vi "Main.vi"(11 "Module Admin":refnum<class "Delacor_lib_QMH_Module Admin.lvclass">) -> ()   [LabVIEW 2020, in "MainUI.lvlib"]
doc: "This template is based off of the Queued Message Handler design pattern and the Queued Message Handler project template that ships with LabVIEW.\n\nThe main difference is that the queue is private to this module and communication between modules is performed via Broadcast and Request events.\n\nRequest events are wrapped in public API methods and are handled in the Event Handling Loop (EHL) of this VI. Any module can register for Broadcast events sent by this module. The EHL generates messages based on user interface actions.\n\nThe Message Handling Loop (MHL) processes messages generated by the EHL, or by other messages. The messages are string values, so new messages can be added easily to the Message Cases case structure in the MHL. Each message cluster can also provide an optional value for Message Data, which is a variant that can be converted to whatever message-specific data is required.\n_____\nBased on Delacor QMH Project Template 4.0.0.47.\n_____\nBased on Delacor QMH Project Template 5.0.0.82."
uses:
  MainUI.lvlib
  <vilib>/Delacor/Delacor QMH/Libraries/Module Admin_class/Delacor_lib_QMH_Module Admin.lvclass
  Module Data--cluster.ctl
  Stop Argument--cluster.ctl
  <vilib>/Delacor/Delacor QMH/Libraries/Message Queue_class/Delacor_lib_QMH_Message Queue.lvclass/Delacor_lib_QMH_Message Queue.ctl
  <vilib>/Delacor/Delacor QMH/Libraries/Module Admin_class/Delacor_lib_QMH_Module Admin.lvclass/Delacor_lib_QMH_Module Admin.ctl
  <vilib>/Delacor/Delacor QMH/Libraries/Message Queue_class/Delacor_lib_QMH_Enqueue Message (Single).vi
  <vilib>/Delacor/Delacor QMH/Libraries/Module Admin_class/Delacor_lib_QMH_Get External Launch.vi
  <vilib>/Waveform/WDTOps.llb/WDT Get XY Value DBL.vi
  <vilib>/Utility/error.llb/Error Cluster From Error Code.vi
  <vilib>/ErrorRing/Error Ring.xnode
  <vilib>/Delacor/Delacor QMH/Libraries/Message Queue_class/Delacor_lib_QMH_Message Queue.lvclass
  Settings Editor/Settings Editor.lvlib
  Acquisition/GetTemperature.lvlib
  Logger/FileLogging.lvlib
panel:
  out "Data":waveform(dbl)[](graph)
  out "Log File Base Path":path
  out "Thermocouple Channel":refnum<k21>
  out "Units\nUnits":i32(ring) items=["degC", "degF", "kelvin", "raw"]
  out "Temperature":dbl
  out "Time Stamp":timestamp
  out "Status":string
  out "Calibrated?":bool
  in  "Calibrate":bool
  in  "Settings":bool
  in  "Start":bool
  in  "Stop":bool
  out "Logger Running?":bool
  out "Settings Editor Running?":bool
  out "Acquisition Running?":bool
  out "error out":errorcluster
  out "version":string
  # "Thermocouple Device Channel Logging"
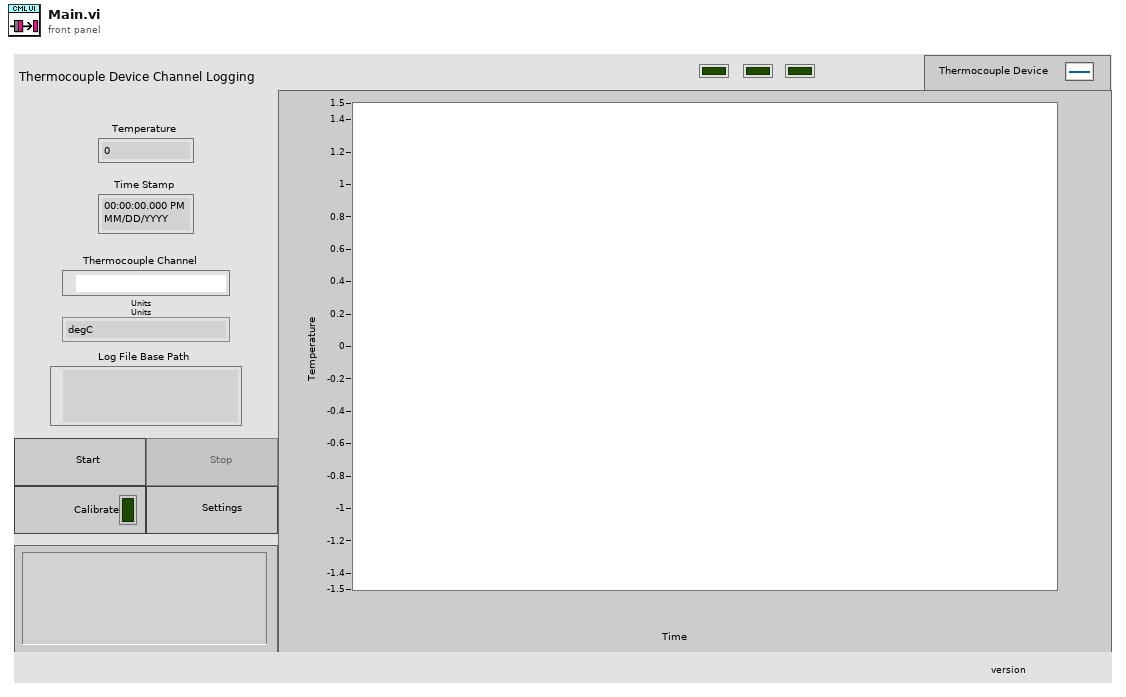
[diagram p1: front panel]
types:
  T1 = typedef "MainUI.lvlib/Request Events--cluster.ctl" = cluster{"Stop Module":refnum<user-event>, "Show Panel":refnum<user-event>, "Hide Panel":refnum<user-event>, "Get Module Execution Status":refnum<user-event>, "Show Diagram":refnum<user-event>}
  T2 = typedef "Settings Editor.lvlib/Broadcast Events--cluster.ctl" = cluster{"Module Did Init":refnum<user-event>, "Status Updated":refnum<user-event>, "Error Reported":refnum<user-event>, "Module Did Stop":refnum<user-event>, "Update Module Execution Status":refnum<user-event>, "Application Settings Updated":refnum<user-event>}
  T3 = typedef "GetTemperature.lvlib/Broadcast Events--cluster.ctl" = cluster{"Module Did Init":refnum<user-event>, "Status Updated":refnum<user-event>, "Error Reported":refnum<user-event>, "Module Did Stop":refnum<user-event>, "Update Module Execution Status":refnum<user-event>, "Acquisition Started":refnum<user-event>, "Acquisition Stopped":refnum<user-event>, "Data Updated":refnum<user-event>, "Device Calibrated":refnum<user-event>}
  T4 = typedef "FileLogging.lvlib/Broadcast Events--cluster.ctl" = cluster{"Module Did Init":refnum<user-event>, "Status Updated":refnum<user-event>, "Error Reported":refnum<user-event>, "Module Did Stop":refnum<user-event>, "Update Module Execution Status":refnum<user-event>, "Logging Stopped":refnum<user-event>, "File Initialized":refnum<user-event>}
  T5 = typedef "MainUI.lvlib/Module Data--cluster.ctl" = cluster{"Status":string, "Measurement UI Controls":cluster{"Start Ref":refnum<vi>, "Stop Ref":refnum<vi>, "Settings Ref":refnum<vi>, "Status Ref":refnum<vi>, "Data Ref":refnum<vi>}}
  T6 = enum32{"invalid lock state", "Not Locked", "Locked (No Password)", "Password-protected"}
  T7 = typedef "MainUI.lvlib/Stop Argument--cluster.ctl" = cluster{"Origin":string, "Exit via Stop Module Req?":bool, "Wait for Module to stop?":bool}
  T8 = enum32{"Invalid", "Standard", "Closed", "Hidden", "Minimized", "Maximized"}
  T9 = typedef "Settings Editor.lvlib/Update Application Settings (Reply Payload)--cluster.ctl" = cluster{"Settings":T10, "Update Settings_error":errorcluster}
  T10 = typedef "Settings Editor.lvlib/Settings--cluster.ctl" = cluster{"Log File Base Path":path, "Analog Input Channel":refnum<k21>, "Units":i32}
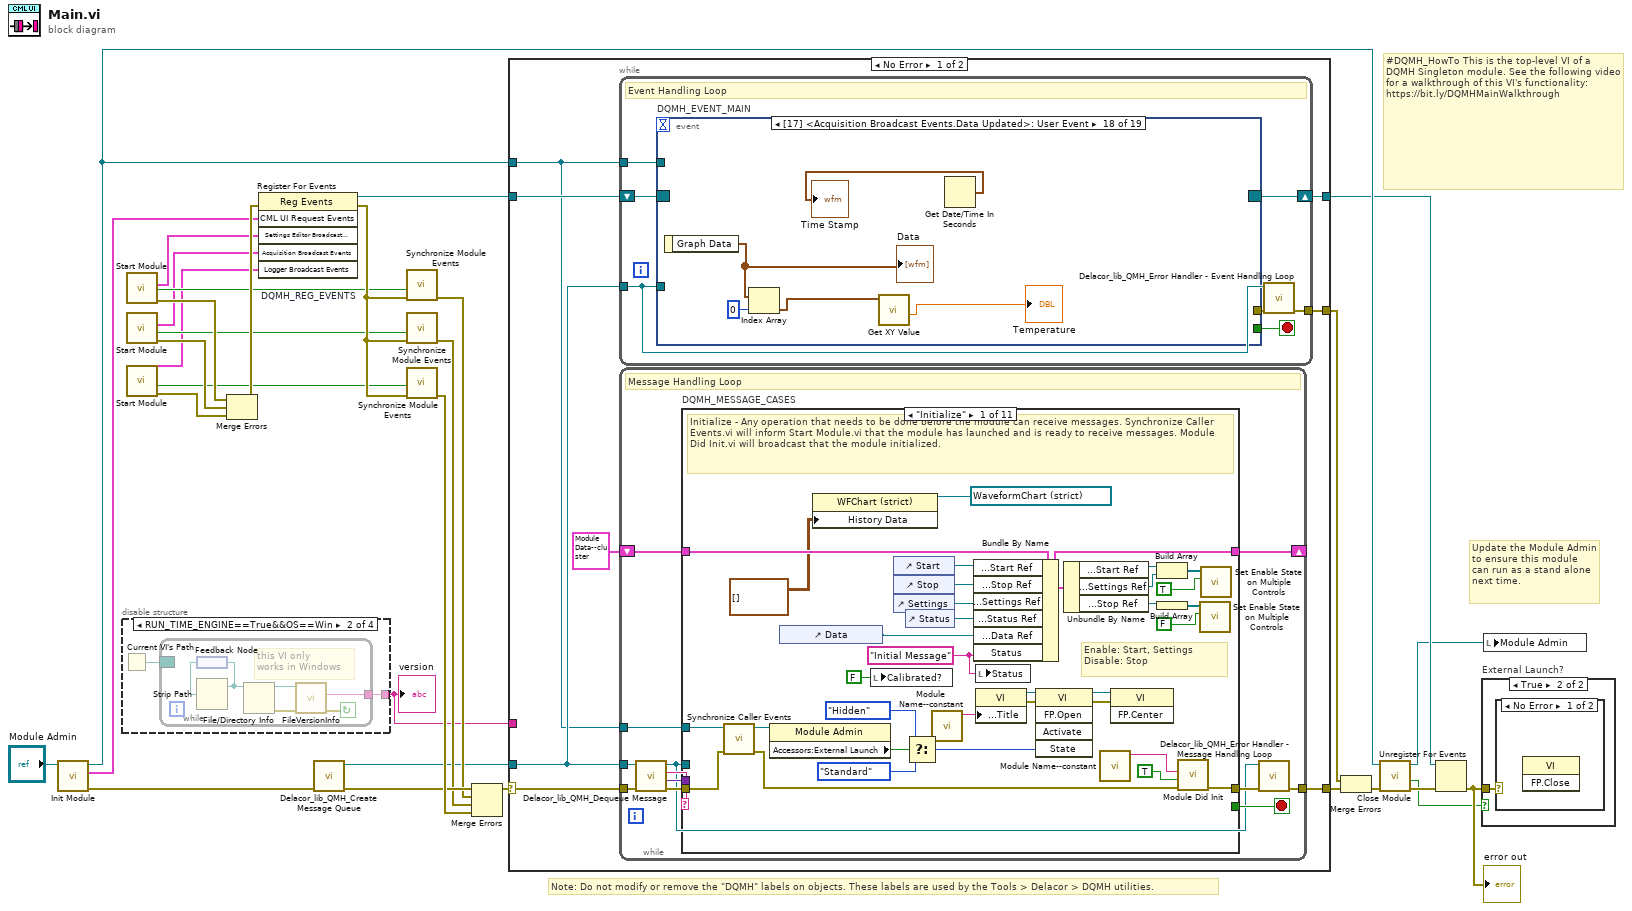
[diagram p0: block diagram]
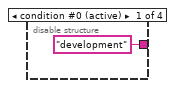
[diagram p2: hidden frame]
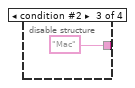
[diagram p3: hidden frame]
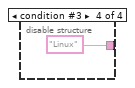
[diagram p4: hidden frame]
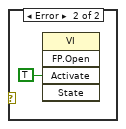
[diagram p6: hidden frame]
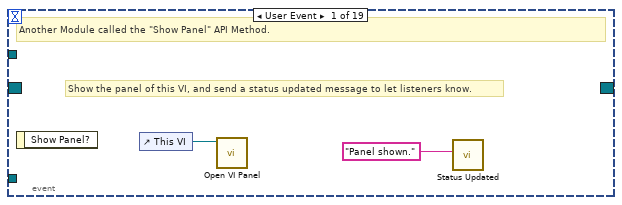
[diagram p7: hidden frame]
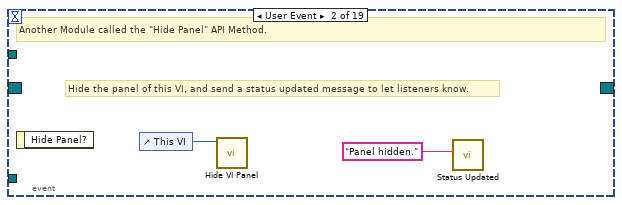
[diagram p8: hidden frame]
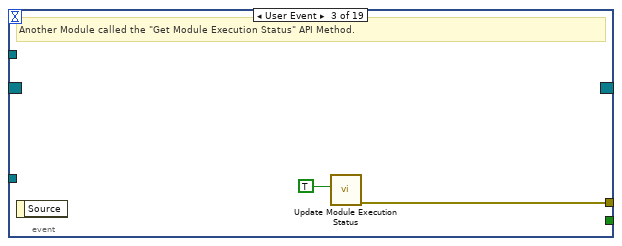
[diagram p9: hidden frame]
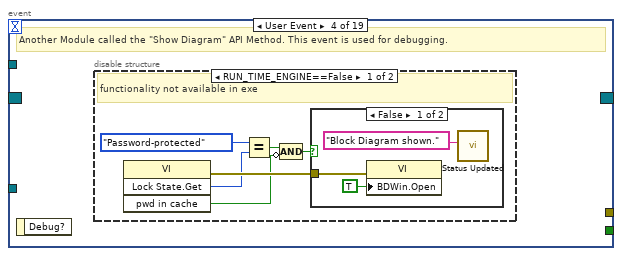
[diagram p10: hidden frame]
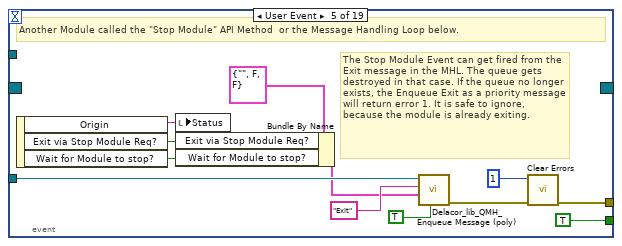
[diagram p13: hidden frame]
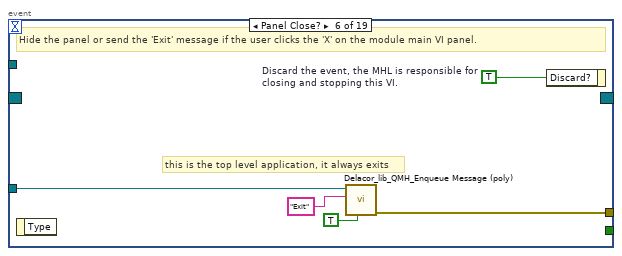
[diagram p14: hidden frame]
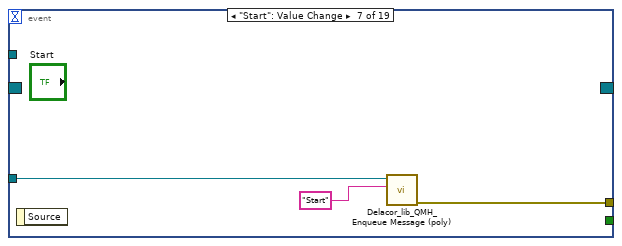
[diagram p15: hidden frame]
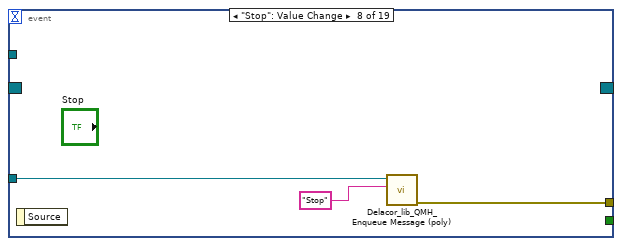
[diagram p16: hidden frame]
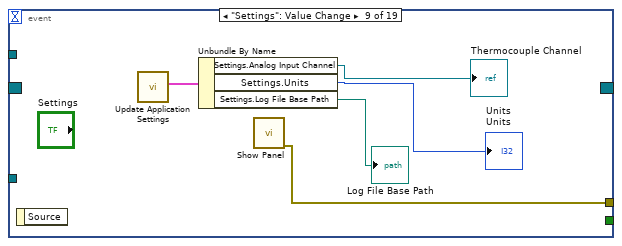
[diagram p17: hidden frame]
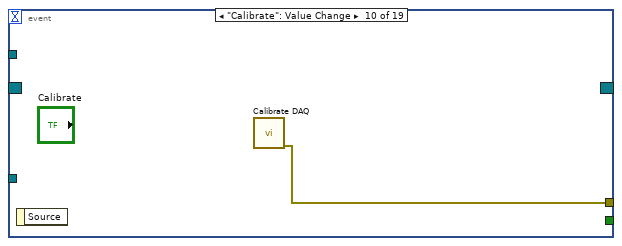
[diagram p18: hidden frame]
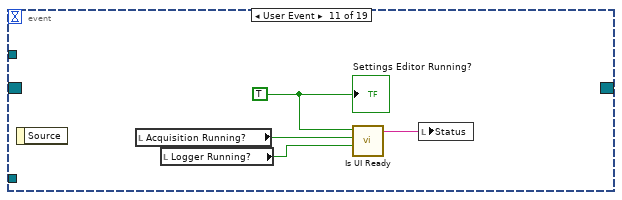
[diagram p19: hidden frame]
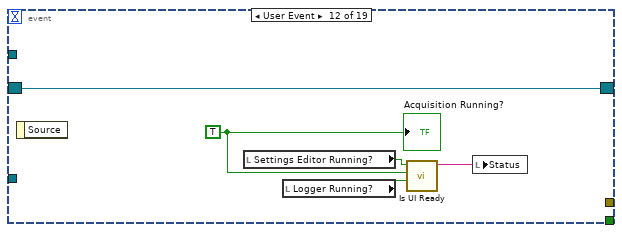
[diagram p20: hidden frame]
diagram:
  # "#DQMH_HowTo This is the top-level VI of a DQMH Singleton module. See the following video for a walkthrough of this VI's functionality: https://bit.ly/DQMHMainWalkthrough"
  # "Note: Do not modify or remove the \"DQMH\" labels on objects. These labels are used by the Tools > Delacor > DQMH utilities."
  # "Update the Module Admin to ensure this module can run as a stand alone next time."
  n1 = call "Init Module.vi"("Singleton Module Admin in"="Module Admin") -> ("error out"=w29:errorcluster, "CML UI Request Events"=w12:T1, "Singleton Module Admin out"=w15:refnum<class "Delacor_lib_QMH_Module Admin.lvclass">)  [unwired: 8 in]
  n2 = disable-structure "Conditional Disable Structure" shown="RUN_TIME_ENGINE==True&&OS==Win" {
    disable-tunnel: ["development" w33 "Mac" "Linux"] -> w1
    frame condition #0 (active) {
    }
    frame condition #1 {
      n3 = Current VI's Path() -> (path=w34:path)
      n4 = while {
        border: w34 -> [_]
        tunnel: [w35] -> w33
        stop <- w39 continue-if-true
        # "this VI only \nworks in Windows"
        n5 = feedback #1() -> (w38:path)
        n6 = Strip Path(path=w38) -> (stripped path=w37:path)  [unwired: 1 out]
        n7 = feedback-in #1(w37) -> ()
        n8 = File/Directory Info(path=w37) -> (path out=w36:path, error out=w40:errorcluster)  [unwired: 1 in, 5 out]
        n9 = call <vilib>:"FileVersionInfo.vi"("error in (no error)"=w40, "Application Path in"=w36) -> ("error out"=w39:errorcluster, "File Version Info"=w35:string)  [unwired: 6 in, 2 out]
      }
    }
    frame condition #2 {
    }
    frame condition #3 {
    }
  }
  "version" <- w1
  n10 = call "Start Module.vi"() -> ("error out"=w20:errorcluster, "Wait for Event Sync?"=w7:bool, "Settings Editor Broadcast Events"=w6:T2)  [unwired: 8 in, 1 out]
  n11 = call "Start Module.vi"() -> ("error out"=w19:errorcluster, "Wait for Event Sync?"=w4:bool, "Acquisition Broadcast Events"=w5:T3)  [unwired: 8 in, 1 out]
  n12 = call "Start Module.vi"() -> ("error out"=w18:errorcluster, "Wait for Event Sync?"=w2:bool, "Logger Broadcast Events"=w3:T4)  [unwired: 8 in, 1 out]
  n13 = Merge Errors(w20, w19, w18) -> (w17:errorcluster)
  n14 = register-events "DQMH_REG_EVENTS"(error in=w17, w12, w6, w5, w3) -> (reference out=w13:refnum<event-registration>, error out=w16:errorcluster)  [unwired: 1 in]
  n15 = call <vilib>:"Delacor_lib_QMH_Create Message Queue.vi"("error in (no error)"=w29) -> ("error out"=w24:errorcluster, "Message Queue"=w11:refnum<class "Delacor_lib_QMH_Message Queue.lvclass">)  [unwired: 9 in]
  n16 = call "Synchronize Module Events.vi"("error in (no error)"=w16, "Wait for Event Sync?"=w7) -> ("error out"=w22:errorcluster)  [unwired: 9 in]
  n17 = call "Synchronize Module Events.vi"("error in (no error)"=w16, "Wait for Event Sync?"=w4) -> ("error out"=w21:errorcluster)  [unwired: 9 in]
  n18 = call "Synchronize Module Events.vi"("error in (no error)"=w16, "Wait for Event Sync?"=w2) -> ("error out"=w31:errorcluster)  [unwired: 9 in]
  n19 = Merge Errors(w24, w22, w21, w31) -> (w23:errorcluster)
  n20 = case shown="No Error" w23 {
    selector: w23 -> [w48 w263]
    tunnel: [w50 w262] -> w30
    tunnel: [w47 w271] -> w14
    tunnel: w13 -> [w45 w271]
    tunnel: w11 -> [w44 w264]
    tunnel: [w49 _] -> w27
    tunnel: w15 -> [w43 w267]
    tunnel: w1 -> [_ _]
    frame No Error {
      n21 = while {
        tunnel: w44 -> [w51]
        shift-right: [w54] -> w47
        shift-left: w45 -> [w55]
        tunnel: [w56] -> w49
        tunnel: w43 -> [w52]
        stop <- w53 stop-if-true
        # "Event Handling Loop"
        n22 = event "DQMH_EVENT_MAIN" shown="[17] <Acquisition Broadcast Events.Data Updated>: User Event" {
          selector: w55 -> [_ _ _ _ _ _ _ _ _ _ _ w110 _ _ _ _ _ _ _]
          dyn-events: [_ _ _ _ _ _ _ _ _ _ _ w110 _ _ _ _ _ _ _] -> w54
          timeout: _ -> [_ _ _ _ _ _ _ _ _ _ _ _ _ _ _ _ _ _ _]
          tunnel: [_ _ _ _ TRUE ("Discard?") _ _ _ _ _ _ _ _ _ _ _ _ _ _] -> w53
          tunnel: w51 -> [_ _ _ _ w80 w87 w90 w93 _ _ _ _ _ _ _ w122 w124 _ _]
          tunnel: [_ _ w63 _ w83 w89 w92 w95 w100 w101 _ _ _ _ w120 _ _ _ _] -> w57
          tunnel: w52 -> [_ _ _ _ _ _ _ _ _ _ _ _ _ _ _ _ _ _ _]
          event User Event {
            # "Show the panel of this VI, and send a status updated message to let listeners know."
            # "Another Module called the \"Show Panel\" API Method."
            n23 = event-data() -> ()  [unwired: 1 in, 1 out]
            n24 = control-ref of="This VI"() -> (w59:refnum<vi>)
            n25 = call "Open VI Panel.vi"("VI"=w59) -> ()  [unwired: 10 in, 1 out]
            n26 = call "Status Updated.vi"("Status"="Panel shown." ("format string")) -> ()  [unwired: 10 in, 1 out]
          }
          event User Event {
            # "Hide the panel of this VI, and send a status updated message to let listeners know."
            # "Another Module called the \"Hide Panel\" API Method."
            n27 = event-data() -> ()  [unwired: 1 in, 1 out]
            n28 = control-ref of="This VI"() -> (w61:refnum<vi>)
            n29 = call "Hide VI Panel.vi"("VI"=w61) -> ()  [unwired: 10 in, 1 out]
            n30 = call "Status Updated.vi"("Status"="Panel hidden." ("format string")) -> ()  [unwired: 10 in, 1 out]
          }
          event User Event {
            # "Another Module called the \"Get Module Execution Status\" API Method."
            n31 = event-data() -> ()  [unwired: 1 in, 1 out]
            n32 = call "Update Module Execution Status.vi"("Running?"=TRUE) -> ("error out"=w63:errorcluster)  [unwired: 10 in]
          }
          event User Event {
            # "Another Module called the \"Show Diagram\" API Method. This event is used for debugging."
            n33 = event-data() -> ()  [unwired: 1 in, 1 out]
            n34 = disable-structure shown="RUN_TIME_ENGINE==False" {
              frame condition #0 (active) {
                # "functionality not available in exe"
                n35 = invoke on="Invoke Node" class="VI" method="Lock State.Get"() -> (error out=w69:errorcluster, "Get Lock State"=w68:T6, "pwd in cache"=w65:bool)  [unwired: 4 in, 1 out]
                n36 = Equal?(x=T6."Password-protected", y=w68) -> (x = y?=w66:bool)
                n37 = Compound Arithmetic op=AND(w66, invert w65) -> (w64:bool)
                n38 = case shown="False" w64 {
                  tunnel: w69 -> [w72 _]
                  frame False {
                    n39 = property on="Property Node" class="VI"(error in=w72, "BDWin.Open"=TRUE ("Block Diagram Window:Open")) -> ()  [unwired: 1 in, 2 out]
                    n40 = call "Status Updated.vi"("Status"="Block Diagram shown." ("format string")) -> ()  [unwired: 10 in, 1 out]
                  }
                  frame True {
                    # "Password-protected VI, and the password is not in the cache. Do not show the diagram."
                  }
                }
              }
              frame condition #1 {
              }
            }
          }
          event User Event {
            # "The Stop Module Event can get fired from the Exit message in the MHL. The queue gets destroyed in that case. If the queue no longer exists, the Enqueue Exit as a priority message will return error 1. It is safe to ignore, because the module is already exiting."
            # "Another Module called the \"Stop Module\" API Method  or the Message Handling Loop below."
            n41 = event-data() -> ("Origin"=w79:string, "Exit via Stop Module Req?"=w75:bool, "Wait for Module to stop?"=w74:bool)  [unwired: 1 in]
            n42 = local write "Status"(w79) -> ()
            n43 = Bundle By Name(cluster=T7 {"Origin"="", "Exit via Stop Module Req?"=FALSE, "Wait for Module to stop?"=FALSE} ("Stop Argument"), "Exit via Stop Module Req?"=w75, "Wait for Module to stop?"=w74) -> (w73:T7)
            n44 = call-poly <vilib>:"Delacor_lib_QMH_Enqueue Message (poly).vi"("Priority Message? (F)"=TRUE, "Message Data"=w73, "Message"="Exit", "Message Queue in"=w80) -> ("error out"=w84:errorcluster)  [unwired: 6 in, 1 out]
            n45 = call <vilib>:"Clear Errors.vi"("error in (no error)"=w84, "specific error code to clear (0: all)"=1) -> ("error out"=w83:errorcluster)  [unwired: 4 in, 1 out]
          }
          event Panel Close? {
            w88 = TRUE  # Discard the event, the MHL is responsible for closing and stopping this VI.
            # "this is the top level application, it always exits"
            # "Hide the panel or send the 'Exit' message if the user clicks the 'X' on the module main VI panel."
            n46 = event-data() -> ()  [unwired: 1 in, 1 out]
            n47 = call-poly <vilib>:"Delacor_lib_QMH_Enqueue Message (poly).vi"("Priority Message? (F)"=TRUE, "Message"="Exit", "Message Queue in"=w87) -> ("error out"=w89:errorcluster)  [unwired: 7 in, 1 out]
            n48 = event-data ("Event Filter Node")("Discard?"=w88) -> ()  [unwired: 1 in, 1 out]
          }
          event "Start": Value Change {
            n49 = event-data() -> ()  [unwired: 1 in, 1 out]
            n50 = call-poly <vilib>:"Delacor_lib_QMH_Enqueue Message (poly).vi"("Message"="Start", "Message Queue in"=w90) -> ("error out"=w92:errorcluster)  [unwired: 8 in, 1 out]
          }
          event "Stop": Value Change {
            n51 = event-data() -> ()  [unwired: 1 in, 1 out]
            n52 = call-poly <vilib>:"Delacor_lib_QMH_Enqueue Message (poly).vi"("Message"="Stop", "Message Queue in"=w93) -> ("error out"=w95:errorcluster)  [unwired: 8 in, 1 out]
          }
          event "Settings": Value Change {
            n53 = event-data() -> ()  [unwired: 1 in, 1 out]
            n54 = call "Update Application Settings.vi"() -> ("Reply Payload"=w99:T9)  [unwired: 9 in, 2 out]
            n55 = Unbundle By Name(w99) -> ("Settings.Analog Input Channel"=→"Thermocouple Channel":refnum<k21>, "Settings.Units"=→"Units\nUnits":i32, "Settings.Log File Base Path"=→"Log File Base Path":path)
            n56 = call "Show Panel.vi"() -> ("error out"=w100:errorcluster)  [unwired: 11 in]
          }
          event "Calibrate": Value Change {
            n57 = event-data() -> ()  [unwired: 1 in, 1 out]
            n58 = call "Calibrate DAQ.vi"() -> ("error out"=w101:errorcluster)  [unwired: 11 in]
          }
          event User Event {
            w103 = TRUE ("Settings Editor Running?")
            n59 = event-data() -> ()  [unwired: 1 in, 1 out]
            n60 = local read "Acquisition Running?"() -> (w105:bool)
            n61 = local read "Logger Running?"() -> (w104:bool)
            n62 = call "Is UI Ready.vi"("Logger Running?"=w104, "Acquisition Running?"=w105, "Settings Editor Running?"=w103) -> ("Status"=w102:string)  [unwired: 8 in]
            n63 = local write "Status"(w102) -> ()
            "Settings Editor Running?" <- w103
          }
          event User Event {
            w108 = TRUE ("Acquisition Running?")
            n64 = event-data() -> ()  [unwired: 1 in, 1 out]
            n65 = local read "Settings Editor Running?"() -> (w107:bool)
            n66 = local read "Logger Running?"() -> (w106:bool)
            n67 = call "Is UI Ready.vi"("Logger Running?"=w106, "Acquisition Running?"=w108, "Settings Editor Running?"=w107) -> ("Status"=w109:string)  [unwired: 8 in]
            n68 = local write "Status"(w109) -> ()
            "Acquisition Running?" <- w108
          }
          event User Event {
            w113 = TRUE ("Logger Running?")
            n69 = event-data() -> ()  [unwired: 1 in, 1 out]
            n70 = local read "Settings Editor Running?"() -> (w112:bool)
            n71 = local read "Acquisition Running?"() -> (w111:bool)
            n72 = call "Is UI Ready.vi"("Logger Running?"=w113, "Acquisition Running?"=w111, "Settings Editor Running?"=w112) -> ("Status"=w114:string)  [unwired: 8 in]
            n73 = local write "Status"(w114) -> ()
            "Logger Running?" <- w113
          }
          event User Event {
            n74 = event-data() -> ("Status"=w115:string)  [unwired: 1 in]
            "Status" <- w115
            n75 = call "Status Updated.vi"("Status"=w115) -> ()  [unwired: 10 in, 1 out]
          }
          event User Event {
            n76 = event-data() -> ("Error"=w120:errorcluster, "Module Name"=w118:string)  [unwired: 1 in, 1 out]
            n77 = Unbundle By Name(w120) -> ("code"=w119:i32)
            n78 = Format Into String(format string="Error %d at %s", w119, w118) -> (resulting string=w117:string)  [unwired: 2 in, 1 out]
            n79 = local write "Status"(w117) -> ()
          }
          event User Event {
            n80 = event-data() -> ()  [unwired: 1 in, 1 out]
            n81 = call-poly <vilib>:"Delacor_lib_QMH_Enqueue Message (poly).vi"("Message"="Acquisition Started Interlocks", "Message Queue in"=w122) -> ()  [unwired: 8 in, 2 out]
          }
          event User Event {
            n82 = event-data() -> ()  [unwired: 1 in, 1 out]
            n83 = call-poly <vilib>:"Delacor_lib_QMH_Enqueue Message (poly).vi"("Message"="Acquisition Stopped Interlocks", "Message Queue in"=w124) -> ()  [unwired: 8 in, 2 out]
          }
          event User Event {
            n84 = event-data() -> ("Graph Data"=w127:waveform(dbl)[])  [unwired: 1 in]
            "Data" <- w127
            n85 = Index Array(array=w127, index=0) -> (element=w126:waveform(dbl))
            n86 = call-poly <vilib>:"Get XY Value.vi"("waveform in"=w126) -> ("Y value"=→"Temperature":dbl)  [unwired: 6 in, 4 out]
            n87 = Get Date/Time In Seconds() -> (seconds since 1Jan1904=→"Time Stamp":timestamp)
          }
          event User Event {
            n88 = event-data() -> ()  [unwired: 1 in, 1 out]
            "Calibrated?" <- TRUE ("Calibrated?")
          }
        }
        n89 = call-dynamic "Delacor_lib_QMH_Error Handler - Event Handling Loop.vi"("error in (no error)"=w57, "Message Queue in"=w51) -> ("dup error in"=w56:errorcluster)  [unwired: 8 in, 1 out]
      }
      n90 = while {
        tunnel: w44 -> [w133]
        shift-right: [w137] -> _
        shift-left: T5 {"Status"="", "Measurement UI Controls"={"Start Ref"=refnum, "Stop Ref"=refnum, "Settings Ref"=refnum, "Status Ref"=refnum, "Data Ref"=refnum}} ("Data Cluster") -> [w138]
        tunnel: w48 -> [w141]
        tunnel: [w139] -> w50
        tunnel: w43 -> [w131]
        stop <- w136 stop-if-true
        # "Message Handling Loop"
        n91 = call-dynamic "Delacor_lib_QMH_Dequeue Message.vi"("error in (no error)"=w141, "Message Queue in"=w133) -> ("error out"=w140:errorcluster, "Message Data"=w134:variant, "Message"=w135:string, "Message Queue out"=w132:refnum<class "Delacor_lib_QMH_Message Queue.lvclass">)  [unwired: 6 in]
        n92 = case "DQMH_MESSAGE_CASES" shown="\"Initialize\"" w135 {
          selector: w135 -> [_ _ _ _ _ _ _ _ _ _ w249]
          tunnel: w132 -> [_ _ _ _ _ _ _ _ w213 w240 _]
          tunnel: w140 -> [w174 w178 w181 w191 w194 w204 w207 w209 w220 w245 w251]
          tunnel: [w172 w178 w180 w191 w193 w204 w206 w209 w216 w229 w252] -> w142
          tunnel: w138 -> [w163 w177 w179 w183 w192 w196 w205 w208 w215 w239 w250]
          tunnel: [w154 w177 w179 w183 w192 w196 w205 w208 w215 w239 w250] -> w137
          tunnel: [_ _ _ _ _ _ _ _ _ w238 _] -> w136
          tunnel: w134 -> [_ _ _ _ _ _ _ _ w214 w237 _]
          tunnel: w131 -> [w164 _ _ _ _ _ _ _ w212 w232 _]
          frame "Initialize" {
            w159 = "Initial Message" ("Initial Message")
            # "Enable: Start, Settings\nDisable: Stop"
            # "Initialize - Any operation that needs to be done before the module can receive messages. Synchronize Caller Events.vi will inform Start Module.vi that the module has launched and is ready to receive messages. Module Did Init.vi will broadcast that the module initialized."
            n93 = call "Synchronize Caller Events.vi"("error in (no error)"=w174, "Singleton Module Admin in"=w164) -> ("error out"=w173:errorcluster, "Singleton Module Admin out"=w160:refnum<class "Delacor_lib_QMH_Module Admin.lvclass">)  [unwired: 8 in]
            n94 = property on="Property Node" class="Module Admin"(reference=w160) -> ("Accessors:External Launch"=w168:bool)  [unwired: 1 in, 2 out]
            n95 = control-ref of="Data"() -> (w145:refnum<vi>)
            n96 = property on="Property Node" class="WFChart (strict)"(reference=refnum<vi> refnum, "History Data"=waveform(dbl)[][] []) -> ()  [unwired: 1 in, 2 out]
            n97 = local write "Calibrated?"(FALSE ("Calibrated?")) -> ()
            n98 = control-ref of="Start"() -> (w158:refnum<vi>)
            n99 = control-ref of="Stop"() -> (w157:refnum<vi>)
            n100 = control-ref of="Settings"() -> (w156:refnum<vi>)
            n101 = control-ref of="Status"() -> (w155:refnum<vi>)
            n102 = Select(t=T8."Hidden" ("State"), s=w168, f=T8."Standard" ("State")) -> (s? t:f=w165:T8)
            n103 = call "Module Name--constant.vi"() -> ("Module Name"=w171:string)  [unwired: 11 in]
            n104 = Bundle By Name(cluster=w163, "Measurement UI Controls.Start Ref"=w158, "Measurement UI Controls.Stop Ref"=w157, "Measurement UI Controls.Settings Ref"=w156, "Measurement UI Controls.Status Ref"=w155, "Measurement UI Controls.Data Ref"=w145, "Status"=w159) -> (w154:T5)
            n105 = local write "Status"(w159) -> ()
            n106 = property on="Property Node" class="VI"("Front Panel.Title"=w171) -> (reference out=w170:refnum<vi>, error out=w176:errorcluster)  [unwired: 2 in]
            n107 = invoke on="Invoke Node" class="VI" method="FP.Open"(reference=w170, error in=w176, "State"=w165) -> (reference out=w169:refnum<vi>, error out=w175:errorcluster)  [unwired: 2 in, 3 out]
            n108 = Unbundle By Name(w154) -> ("Measurement UI Controls.Start Ref"=w153:refnum<vi>, "Measurement UI Controls.Settings Ref"=w152:refnum<vi>, "Measurement UI Controls.Stop Ref"=w149:refnum<vi>)
            n109 = call "Module Name--constant.vi"() -> ("Module Name"=w161:string)  [unwired: 11 in]
            n110 = invoke on="Invoke Node" class="VI" method="FP.Center"(reference=w169, error in=w175) -> ()  [unwired: 1 in, 3 out]
            n111 = Build Array(w153, w152) -> (w151:refnum<vi>[])
            n112 = Build Array(w149) -> (w148:refnum<vi>[])
            n113 = call "Module Did Init.vi"("error in (no error)"=w173, "Initialized?"=TRUE, "Origin"=w161) -> ("error out"=w172:errorcluster)  [unwired: 8 in]
            n114 = call "Set Enable State on Multiple Controls.vi"("Enable?"=FALSE, "Controls"=w148) -> ()  [unwired: 10 in]
            n115 = call "Set Enable State on Multiple Controls.vi"("Enable?"=TRUE, "Controls"=w151) -> ()  [unwired: 10 in]
          }
          frame "--- Module Specific ---" {
            # "Separator -- The following cases handle messages specific to this Module."
          }
          frame "Start" {
            # "End user pressed Start button. Need to request for Acquisition to start acquiring and for Logger to start logging."
            n116 = call "Initialize File.vi"("error in (no error)"=w181) -> ("error out"=w182:errorcluster)  [unwired: 8 in, 2 out]
            n117 = call "Start Acquiring.vi"("error in (no error)"=w182) -> ("error out"=w180:errorcluster)  [unwired: 8 in, 2 out]
          }
          frame "Acquisition Started Interlocks" {
            # "Enable: Stop\nDisable: Start, Settings"
            n118 = Unbundle By Name(w183) -> ("Measurement UI Controls.Stop Ref"=w190:refnum<vi>, "Measurement UI Controls.Start Ref"=w185:refnum<vi>, "Measurement UI Controls.Settings Ref"=w184:refnum<vi>)
            n119 = Build Array(w190) -> (w189:refnum<vi>[])
            n120 = Build Array(w185, w184) -> (w186:refnum<vi>[])
            n121 = call "Set Enable State on Multiple Controls.vi"("Enable?"=TRUE, "Controls"=w189) -> ()  [unwired: 10 in]
            n122 = call "Set Enable State on Multiple Controls.vi"("Enable?"=FALSE, "Controls"=w186) -> ()  [unwired: 10 in]
          }
          frame "Stop" {
            # "End user pressed Stop button. Need to request for Acquisition to stop acquiring and for Logger to stop logging."
            n123 = call "Stop Acquiring.vi"("error in (no error)"=w194) -> ("error out"=w195:errorcluster)  [unwired: 10 in]
            n124 = call "Stop Logging.vi"("error in (no error)"=w195) -> ("error out"=w193:errorcluster)  [unwired: 10 in]
          }
          frame "Acquisition Stopped Interlocks" {
            # "Enable: Start, Settings\nDisable: Stop"
            n125 = Unbundle By Name(w196) -> ("Measurement UI Controls.Stop Ref"=w201:refnum<vi>, "Measurement UI Controls.Start Ref"=w200:refnum<vi>, "Measurement UI Controls.Settings Ref"=w199:refnum<vi>)
            n126 = Build Array(w201) -> (w203:refnum<vi>[])
            n127 = Build Array(w200, w199) -> (w198:refnum<vi>[])
            n128 = call "Set Enable State on Multiple Controls.vi"("Enable?"=FALSE, "Controls"=w203) -> ()  [unwired: 10 in]
            n129 = call "Set Enable State on Multiple Controls.vi"("Enable?"=TRUE, "Controls"=w198) -> ()  [unwired: 10 in]
          }
          frame "---Copy This Frame---" {
            # "Duplicate this frame when creating new messages.  Change this comment in the duplicated frame to describe this message."
            n130 = Merge Errors(w207) -> (w206:errorcluster)
          }
          frame "--- Exit and Error Handling---" {
            # "Separator - The following cases handle errors and exit messages."
          }
          frame "Error" {
            # "Error - Check the error message data and respond accordingly. This message is sent by the \"Error Handler\" VIs at the end of each loop in this application."
            n131 = property on="Property Node" class="Module Admin"(reference=w212) -> ("Accessors:External Launch"=w211:bool)  [unwired: 1 in, 2 out]
            n132 = Variant To Data(error in=w220, type=errorcluster {"status"=FALSE, "code"=0, "source"=""} ("error constant"), Variant=w214) -> (data=w221:errorcluster, error out=w218:errorcluster)
            n133 = call "Module Name--constant.vi"() -> ("Module Name"=w210:string)  [unwired: 11 in]
            n134 = call "Error Reported.vi"("Additional Information"=w210, "Error"=w221) -> ()  [unwired: 9 in, 1 out]
            n135 = case shown="False" w211 {
              tunnel: [w226 _] -> w217
              tunnel: w213 -> [w224 _]
              tunnel: w221 -> [w225 _]
              frame False {
                # "If the module is running standalone, then pop up an error dialog and call the \"Exit\" message."
                n136 = call <vilib>:"Simple Error Handler.vi"("error in (no error)"=w225) -> ()  [unwired: 4 in, 5 out]
                n137 = call-poly <vilib>:"Delacor_lib_QMH_Enqueue Message (poly).vi"("Priority Message? (F)"=TRUE, "Message"="Exit", "Message Queue in"=w224) -> ("error out"=w226:errorcluster)  [unwired: 7 in, 1 out]
              }
              frame True {
                # "If the module was launched externally, calling the Error Reported broadcast VI is the only action performed by the \"Error\" message. The module's caller can then process the error appropriately."
              }
            }
            n138 = Merge Errors(w218, w217) -> (w216:errorcluster)
            n139 = local write "error out"(w216) -> ()
          }
          frame "Exit" {
            w231 = TRUE ("Wait for Module to Stop? (F)")
            w236 = 91  # 91: not all Exit messages will have an argument
            w238 = TRUE  # Stop the VI
            # "DAQ and LOG modules use the settings editor. CML UI module waits for both modules to completely stop before stopping the settings editor."
            # "Release the message queue reference"
            # "Exit - Exit the application."
            n140 = Variant To Data(error in=w245, type=T7 {"Origin"="", "Exit via Stop Module Req?"=FALSE, "Wait for Module to stop?"=FALSE} ("Stop Argument"), Variant=w237) -> (data=w234:T7, error out=w242:errorcluster)
            n141 = call <vilib>:"Clear Errors.vi"("error in (no error)"=w242, "specific error code to clear (0: all)"=w236) -> ("error out"=w244:errorcluster)  [unwired: 4 in, 1 out]
            n142 = control-ref of="This VI"() -> (w233:refnum<vi>)
            n143 = call "Module Name--constant.vi"() -> ("Module Name"=w230:string)  [unwired: 11 in]
            n144 = call "Handle Exit.vi"("Stop Argument"=w234, "Admin in"=w232, "VI reference"=w233) -> ("error out"=w241:errorcluster)  [unwired: 7 in, 1 out]
            n145 = call "Stop Module.vi"("Wait for Module to Stop? (F)"=w231, "Origin"=w230) -> ("error out"=w228:errorcluster)  [unwired: 9 in]
            n146 = call "Stop Module.vi"("Wait for Module to Stop? (F)"=w231, "Origin"=w230) -> ("error out"=w227:errorcluster)  [unwired: 9 in]
            n147 = call-dynamic "Delacor_lib_QMH_Release Message Queue.vi"("error in (no error)"=w244, "Message Queue"=w240) -> ("error out"=w243:errorcluster)  [unwired: 9 in]
            n148 = Merge Errors(w228, w227) -> (w246:errorcluster)
            n149 = Merge Errors(w243, w241) -> (w229:errorcluster)
            n150 = call <vilib>:"Clear Errors.vi"("error in (no error)"=w246) -> ("error out"=w247:errorcluster)  [unwired: 5 in, 1 out]
            n151 = call "Stop Module.vi"("error in (no error)"=w247, "Wait for Module to Stop? (F)"=w231, "Origin"=w230) -> ()  [unwired: 8 in, 1 out]
          }
          frame Default {
            # "'Default' case only runs if there is a message that isn't defined in any of the other cases.  Output a programming error."
            n152 = call "Module Name--constant.vi"() -> ("Module Name"=w248:string)  [unwired: 11 in]
            n153 = xnode ("Error Ring")("parameter 0"=w249, "parameter 1"=w248) -> ("error out"=w253:errorcluster)
            n154 = Merge Errors(w251, w253) -> (w252:errorcluster)
          }
        }
        n155 = call-dynamic "Delacor_lib_QMH_Error Handler - Message Handling Loop.vi"("error in (no error)"=w142, "Message Queue in"=w132) -> ("dup error in"=w139:errorcluster)  [unwired: 8 in, 1 out]
      }
    }
    frame Error {
      w266 = TRUE ("Wait for Module to Stop? (F)")
      # "Synchronize Caller Events.vi will inform Start Module.vi that the module has launched and will let the code calling Start Module.vi register for broadcasts and would permit the caller receive the broadcast that an error occurred at launch time."
      n156 = call-dynamic "Delacor_lib_QMH_Release Message Queue.vi"("error in (no error)"=w263, "Message Queue"=w264) -> ("error out"=w262:errorcluster)  [unwired: 9 in]
      n157 = call "Synchronize Caller Events.vi"("Singleton Module Admin in"=w267) -> ("error out"=w272:errorcluster)  [unwired: 9 in, 1 out]
      n158 = call "Module Name--constant.vi"() -> ("Module Name"=w270:string)  [unwired: 11 in]
      n159 = call "Module Name--constant.vi"() -> ("Module Name"=w265:string)  [unwired: 11 in]
      n160 = call "Stop Module.vi"("Wait for Module to Stop? (F)"=w266, "Origin"=w265) -> ()  [unwired: 9 in, 1 out]
      n161 = call "Stop Module.vi"("Wait for Module to Stop? (F)"=w266, "Origin"=w265) -> ()  [unwired: 9 in, 1 out]
      n162 = call "Stop Module.vi"("Wait for Module to Stop? (F)"=w266, "Origin"=w265) -> ()  [unwired: 9 in, 1 out]
      n163 = Format Into String(format string="An error occurred during initialization. %s is no longer running.", w270) -> (resulting string=w268:string)  [unwired: 2 in, 1 out]
      n164 = Merge Errors(w262, w272) -> (w273:errorcluster)
      n165 = call "Error Reported.vi"("Additional Information"=w268, "Error"=w273) -> ()  [unwired: 9 in, 1 out]
    }
  }
  n166 = Merge Errors(w27, w30) -> (w26:errorcluster)
  n167 = call "Close Module.vi"("error in (no error)"=w26, "Module Admin in"=w15) -> ("error out"=w28:errorcluster, "External Launch"=w8:bool, "Module Admin out"=w9:refnum<class "Delacor_lib_QMH_Module Admin.lvclass">)  [unwired: 7 in]
  n168 = Unregister For Events(event registration refnum=w14, error in=w28) -> (error out=w25:errorcluster)
  "error out" <- w25
  n169 = case "External Launch?" shown="True" w8 {
    tunnel: w25 -> [_ w274]
    frame False {
    }
    frame True {
      n170 = case shown="No Error" w274 {
        frame No Error {
          n171 = invoke class="VI" method="FP.Close"() -> ()  [unwired: 3 in, 3 out]
        }
        frame Error {
          n172 = invoke on="Invoke Node" class="VI" method="FP.Open"("Activate"=TRUE ("Activate?")) -> ()  [unwired: 4 in, 5 out]
        }
      }
    }
  }
  n173 = local write "Module Admin"(w9) -> ()
